vi "PWM output.vi"() -> ()   [LabVIEW 2009, in "MicroDAQ.lvlib"]
uses:
  <instrlib>/MicroDAQ/MicroDAQ.lvlib
  <instrlib>/MicroDAQ/Tools/PWM channel.ctl
  <instrlib>/MicroDAQ/Channel/PWM/PWM Configure.vi
  <instrlib>/MicroDAQ/Channel/PWM/Create.vi
  <instrlib>/MicroDAQ/Channel/PWM/PWM.lvclass
panel:
  in  "IP address":string="10.10.1.1"
  in  "period [us]":u32=1000 min=2 max=500000
  in  "active LOW":u8 max=1
  in  "channel B duty":sgl=50.0
  in  "channel A duty":sgl=50.0
  in  "PWM module":T1=enum."PWM1"
  in  "channel A duty process":sgl=50.0
  in  "channel B duty process":sgl=50.0
  in  "Stop":bool
  # "Device settings"
  # "Channel Init Settings"
  # "Write Setting"
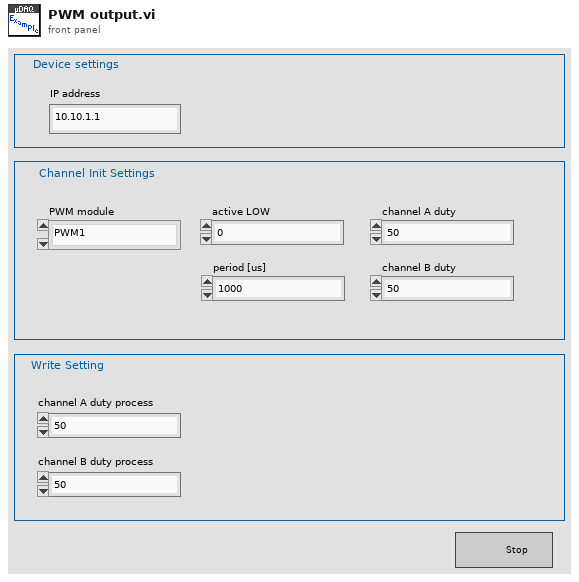
[diagram p1: front panel]
types:
  T1 = typedef "MicroDAQ.lvlib/PWM channel.ctl" = enum8{"None", "PWM1", "PWM2", "PWM3"}
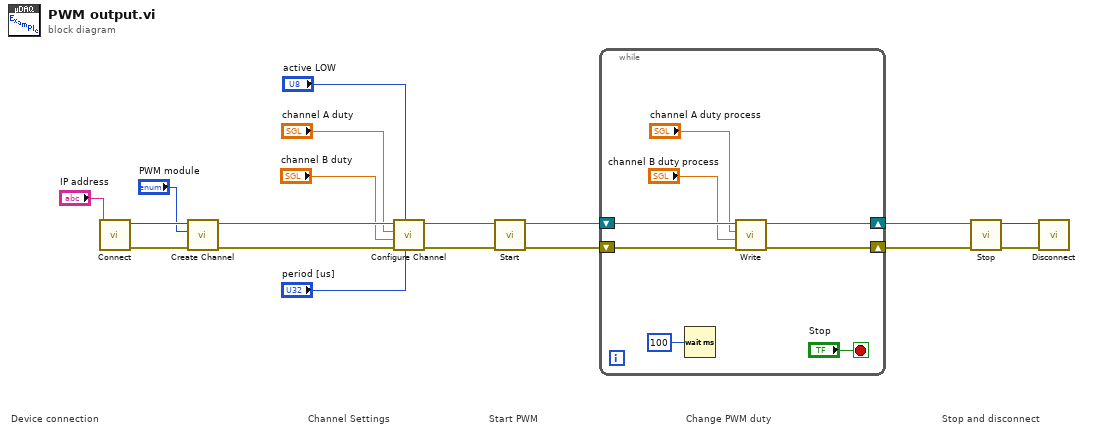
[diagram p0: block diagram]
diagram:
  # "Start PWM"
  # "Device connection"
  # "Change PWM duty"
  # "Stop and disconnect"
  # "Channel Settings"
  n1 = call <instrlib>:"Connect.vi"("IP address"="IP address") -> ("error out"=w17:errorcluster, "connection ID"=w18:i32)  [unwired: 9 in]
  n2 = call-poly <instrlib>:"Create Channel.vi"("error in (no error)"=w17, "PWM module"="PWM module", "connection ID"=w18) -> ("error out"=w11:errorcluster, "MicroDAQ.lvlib:PWM.lvclass"=w12:refnum<class "PWM.lvclass">)  [unwired: 7 in]
  n3 = call-poly <instrlib>:"Configure Channel.vi"("period [ms]"="period [us]", "active LOW"="active LOW", "error in (no error)"=w11, "channel B duty"="channel B duty", "channel A duty"="channel A duty", "Task in"=w12) -> ("error out"=w2:errorcluster, "Task out"=w4:refnum<class "PWM.lvclass">)  [unwired: 4 in]
  n4 = call-dynamic "Start.vi"("error in (no error)"=w2, "Task in"=w4) -> ("error out"=w1:errorcluster, "Task out"=w3:refnum<class "PWM.lvclass">)  [unwired: 8 in]
  n5 = while {
    shift-right: [w22] -> w6
    shift-left: w3 -> [w26]
    shift-right: [w21] -> w5
    shift-left: w1 -> [w25]
    stop <- "Stop" stop-if-true
    n6 = Wait (ms)(milliseconds to wait=u32 100) -> ()  [unwired: 1 out]
    n7 = call-poly <instrlib>:"Write.vi"("error in (no error)"=w25, "channel B duty"="channel B duty process", "channel A duty"="channel A duty process", "Task in"=w26) -> ("error out"=w21:errorcluster, "Task out"=w22:refnum<class "PWM.lvclass">)  [unwired: 6 in]
  }
  n8 = call-dynamic "Stop.vi"("error in (no error)"=w5, "Task in"=w6) -> ("error out"=w14:errorcluster, "connection ID"=w15:i32)  [unwired: 8 in]
  n9 = call <instrlib>:"Disconnect.vi"("error in (no error)"=w14, "connection ID"=w15) -> ()  [unwired: 9 in, 1 out]
